vi "configure operation.vi"(7 "tag bus configurable plugin module configuration":refnum<class "PID Module configuration.lvclass">, 8 "error in":errorcluster, 10 "line item in":T1={"Loop ID"="", "Tags"={"Setpoint"="", "Process Variable"="", "Output"=""}, "Gains"={"P"=1.0, "I"=0.01, "D"=0.0}, "Range"={"High"=100.0, "Low"=-100.0}}, 11 "engine configuration":refnum<class "engine configuration.lvclass">) -> (0 "error out":errorcluster, 1 "success":bool, 2 "PID Loop out":T1={"Loop ID"="", "Tags"={"Setpoint"="", "Process Variable"="", "Output"=""}, "Gains"={"P"=1.0, "I"=0.01, "D"=0.0}, "Range"={"High"=100.0, "Low"=-100.0}}, 5 "changed":bool)   [LabVIEW 2014, in "PID Module editor node.lvclass"]
uses:
  PID Module editor node.lvclass
  PID array element.ctl
  <vilib>/NI/Module Execution Interface/Engine Configuration/engine configuration.lvclass
  module/configuration/PID Module configuration.lvclass
panel:
  in  "Range":cluster{"High":dbl, "Low":dbl}
  in  "Gains":cluster{"P":dbl, "I":dbl, "D":dbl}
  in  "Output":i32(listbox)
  in  "Process Variable":i32(listbox)
  out "errors":string
  in  "Setpoint":i32(listbox)
  in  "PID Loop Name":string
  in  "cancel":bool
  in  "ok":bool
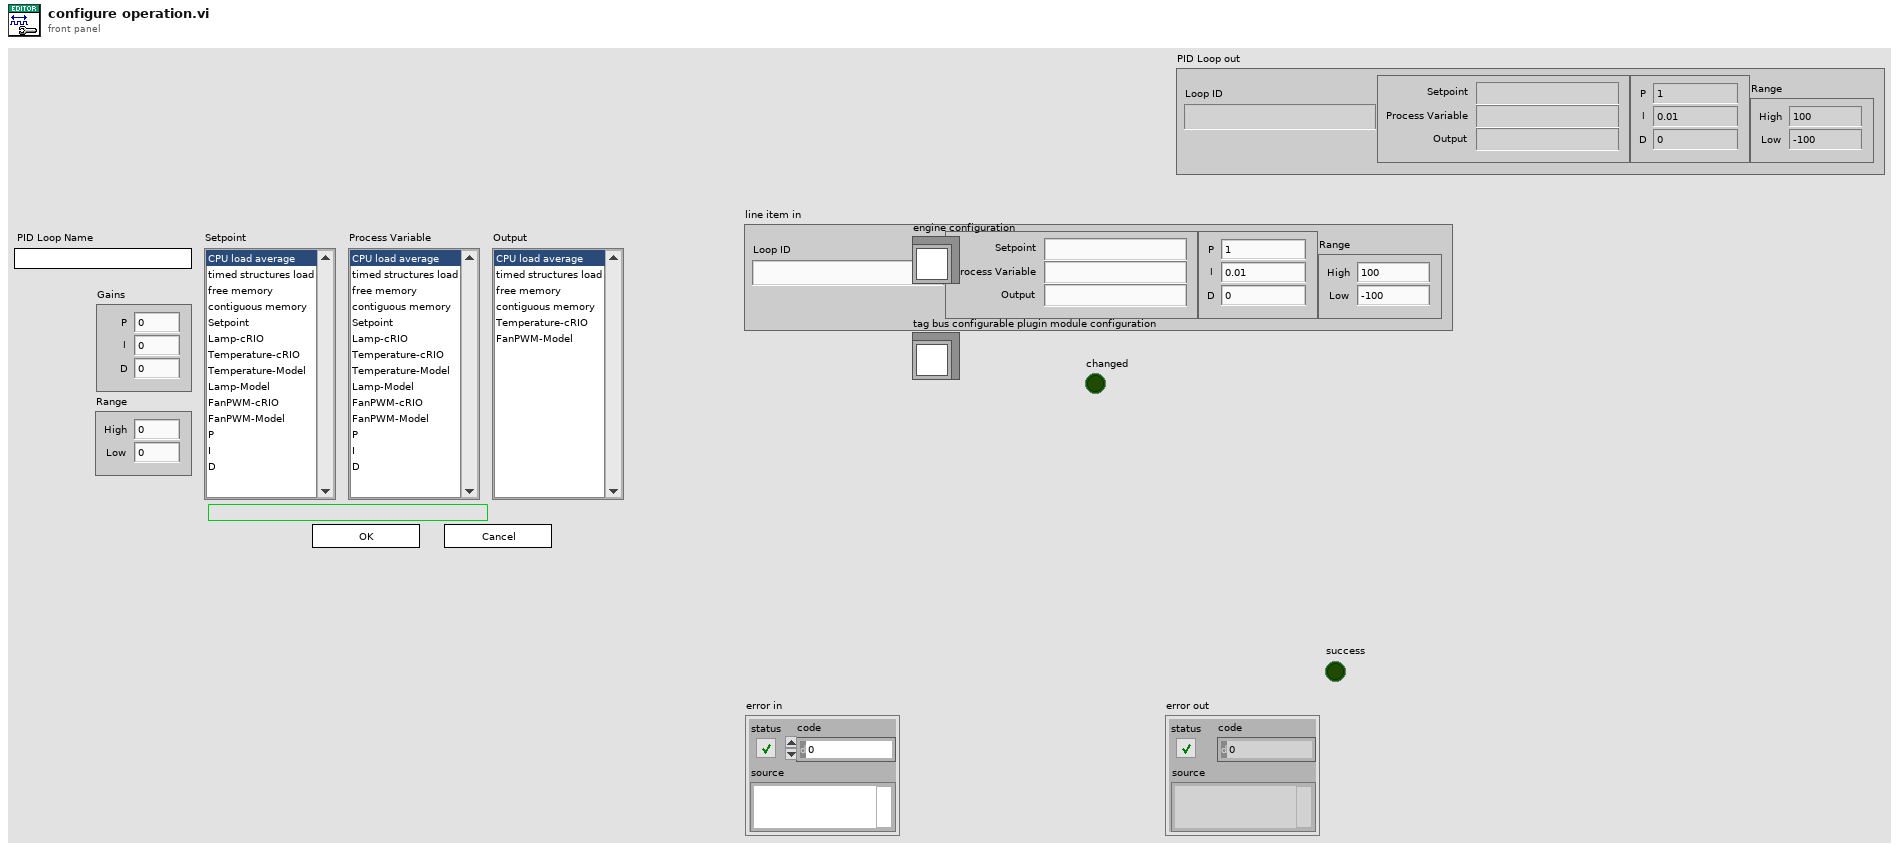
[diagram p1: front panel]
types:
  T1 = typedef "PID Module editor node.lvclass/PID array element.ctl" = cluster{"Loop ID":string, "Tags":cluster{"Setpoint":string, "Process Variable":string, "Output":string}, "Gains":cluster{"P":dbl, "I":dbl, "D":dbl}, "Range":cluster{"High":dbl, "Low":dbl}}
  T2 = enum32{"Invalid", "Standard", "Closed", "Hidden", "Minimized", "Maximized"}
  T3 = enum32{"Invalid", "Default", "Floating", "Floating/Auto-Hide", "Modal"}
  T4 = enum8{"Enabled", "Disabled", "Disabled and Grayed Out"}
  T5 = enum32{"invalid app kind", "Development System", "Run Time System", "Student Edition", "Embedded LabVIEW", "Evaluation", "Custom"}
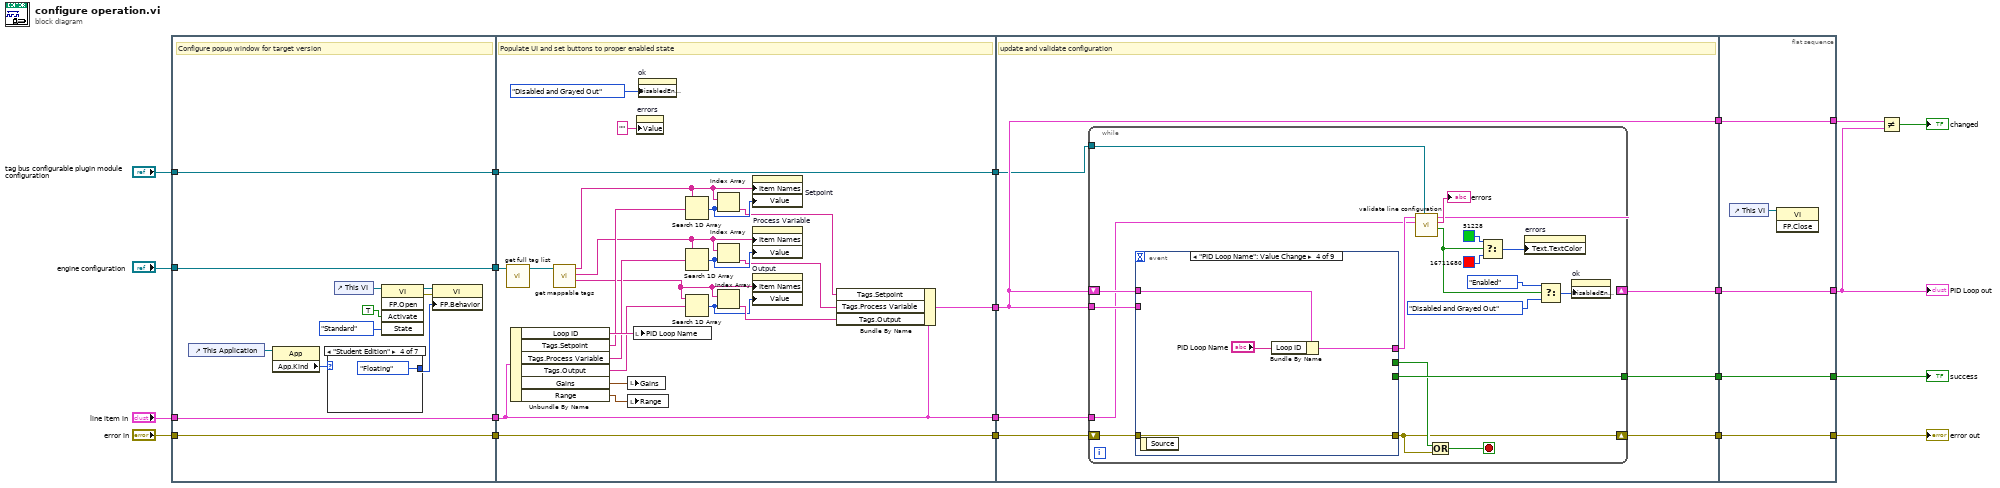
[diagram p0: block diagram]
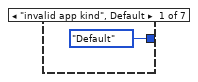
[diagram p2: hidden frame]
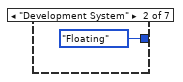
[diagram p3: hidden frame]
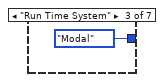
[diagram p4: hidden frame]
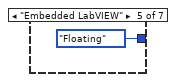
[diagram p5: hidden frame]
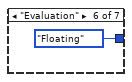
[diagram p6: hidden frame]
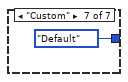
[diagram p7: hidden frame]
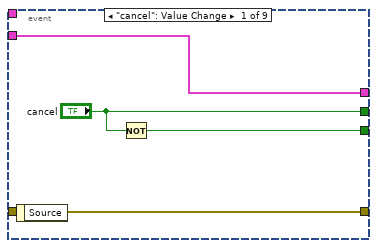
[diagram p8: hidden frame]
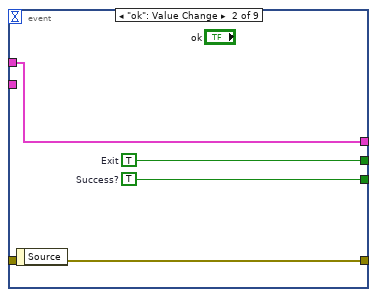
[diagram p9: hidden frame]
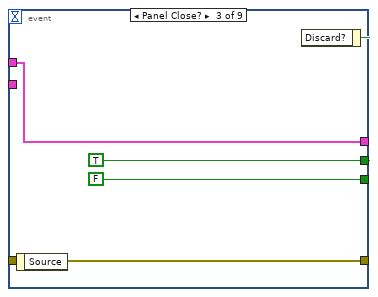
[diagram p10: hidden frame]
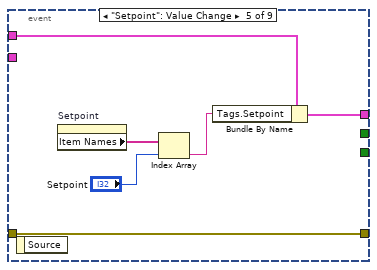
[diagram p11: hidden frame]
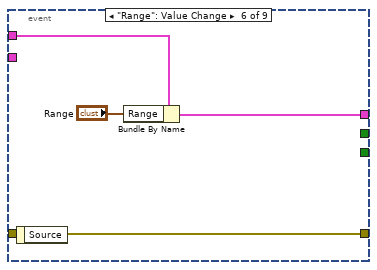
[diagram p12: hidden frame]
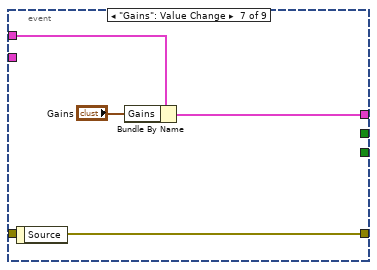
[diagram p13: hidden frame]
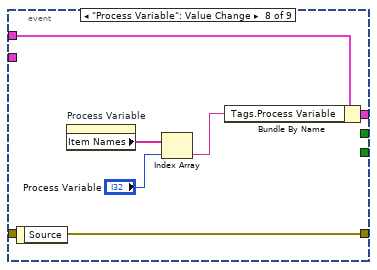
[diagram p14: hidden frame]
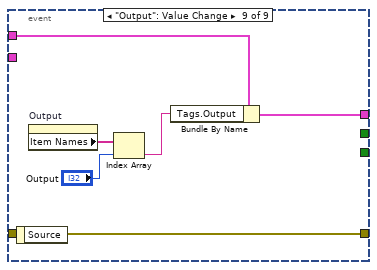
[diagram p15: hidden frame]
diagram:
  n1 = flat-sequence {
    tunnel: "line item in" -> [w32]
    tunnel: "error in" -> [w33]
    tunnel: [w33] -> w10
    tunnel: [w32] -> w9
    tunnel: [w23] -> w7
    tunnel: "engine configuration" -> [w23]
    tunnel: [w22] -> w4
    tunnel: "tag bus configurable plugin module configuration" -> [w22]
    tunnel: w10 -> [w62]
    tunnel: w9 -> [w52]
    tunnel: [w61] -> w8
    tunnel: w7 -> [w47]
    tunnel: [w63] -> w5
    tunnel: w4 -> [w63]
    tunnel: [w62] -> w2
    tunnel: [w52] -> w1
    tunnel: [w69] -> w14
    tunnel: [w68] -> w13
    tunnel: [w67] -> w12
    tunnel: [w66] -> w11
    tunnel: w8 -> [w66]
    tunnel: w5 -> [w65]
    tunnel: w2 -> [w70]
    tunnel: w1 -> [w64]
    tunnel: [w133] -> w15
    tunnel: [w134] -> w18
    tunnel: [w135] -> w19
    tunnel: [w136] -> w20
    tunnel: w14 -> [w136]
    tunnel: w13 -> [w135]
    tunnel: w12 -> [w134]
    tunnel: w11 -> [w133]
    frame #0 {
      # "Configure popup window for target version"
      n2 = control-ref of="This Application"() -> (w26:refnum<vi>)
      n3 = property class="App"(reference=w26) -> ("App.Kind"=w25:T5)  [unwired: 1 in, 2 out]
      n4 = case shown="\"Student Edition\"" w25 {
        tunnel: [T3."Default" ("Front Panel Window:Behavior") T3."Floating" ("Front Panel Window:Behavior") T3."Modal" ("Front Panel Window:Behavior") T3."Floating" ("Front Panel Window:Behavior") T3."Floating" ("Front Panel Window:Behavior") T3."Floating" ("Front Panel Window:Behavior") T3."Default" ("Front Panel Window:Behavior")] -> w24
        frame "invalid app kind", Default {
        }
        frame "Development System" {
        }
        frame "Run Time System" {
        }
        frame "Student Edition" {
        }
        frame "Embedded LabVIEW" {
        }
        frame "Evaluation" {
        }
        frame "Custom" {
        }
      }
      n5 = control-ref of="This VI"() -> (w27:refnum<vi>)
      n6 = invoke class="VI" method="FP.Open"(reference=w27, "Activate"=TRUE ("Activate?"), "State"=T2."Standard") -> (reference out=w30:refnum<vi>, error out=w31:errorcluster)  [unwired: 2 in, 3 out]
      n7 = property class="VI"(reference=w30, error in=w31, "FP.Behavior"=w24) -> ()  [unwired: 2 out]
    }
    frame #1 {
      # "Populate UI and set buttons to proper enabled state"
      n8 = call <vilib>:"get full tag list.vi"("engine configuration in"=w47) -> ("engine configuration out"=w44:refnum<class "engine configuration.lvclass">)  [unwired: 9 in, 1 out]
      n9 = Unbundle By Name(w52) -> ("Loop ID"=w58:string, "Tags.Setpoint"=w55:string, "Tags.Process Variable"=w54:string, "Tags.Output"=w53:string, "Gains"=w56:cluster{"P":dbl, "I":dbl, "D":dbl}, "Range"=w57:cluster{"High":dbl, "Low":dbl})
      n10 = call "get mappable tags.vi"("engine configuration in"=w44) -> ("Output Tags"=w41:string[], "Process Variable Tags"=w42:string[], "Setpoint Tags"=w43:string[])  [unwired: 8 in]
      n11 = local write "Gains"(w56) -> ()
      n12 = local write "Range"(w57) -> ()
      n13 = local write "PID Loop Name"(w58) -> ()
      n14 = property on="errors" class="Str"("Value"="" ("errors")) -> ()  [unwired: 2 in, 2 out]
      n15 = property on="ok" class="Bool"("DisabledEnum"=T4."Disabled and Grayed Out" ("Disabled")) -> ()  [unwired: 2 in, 2 out]
      n16 = Search 1D Array(1D array=w43, element=w55) -> (index of element=w51:i32)  [unwired: 1 in]
      n17 = Search 1D Array(1D array=w42, element=w54) -> (index of element=w50:i32)  [unwired: 1 in]
      n18 = Search 1D Array(1D array=w41, element=w53) -> (index of element=w48:i32)  [unwired: 1 in]
      n19 = Index Array(array=w43, index=w51) -> (element=w46:string)
      n20 = Index Array(array=w42, index=w50) -> (element=w45:string)
      n21 = Index Array(array=w41, index=w48) -> (element=w49:string)
      n22 = property on="Setpoint" class="LstBox (strict)"("Item Names"=w43, "Value"=w51) -> ()  [unwired: 2 in, 2 out]
      n23 = property on="Process Variable" class="LstBox (strict)"("Item Names"=w42, "Value"=w50) -> ()  [unwired: 2 in, 2 out]
      n24 = property on="Output" class="LstBox (strict)"("Item Names"=w41, "Value"=w48) -> ()  [unwired: 2 in, 2 out]
      n25 = Bundle By Name(cluster=w52, "Tags.Setpoint"=w46, "Tags.Process Variable"=w45, "Tags.Output"=w49) -> (w61:T1)
    }
    frame #2 {
      # "update and validate configuration"
      n26 = while {
        shift-right: [w85] -> w68
        shift-left: w70 -> [w89]
        tunnel: [w88] -> w69
        shift-right: [w77] -> w67
        shift-left: w66 -> [w80]
        tunnel: w66 -> [w72]
        tunnel: w65 -> [w81]
        tunnel: w64 -> [w71]
        stop <- w86 stop-if-true
        n27 = event shown="[3] \"PID Loop Name\": Value Change" {
          selector: _ -> [_ _ _ _ _ _ _ _ _]
          dyn-events: _ -> [_ _ _ _ _ _ _ _ _]
          timeout: _ -> [_ _ _ _ _ _ _ _ _]
          tunnel: w89 -> [w93 w97 w101 w105 w106 w115 w119 w120 w127]
          tunnel: [w93 w97 w101 w105 w106 w115 w119 w120 w127] -> w85
          tunnel: [w92 w94 FALSE _ _ _ _ _ _] -> w88
          tunnel: ["cancel" w95 w99 _ _ _ _ _ _] -> w87
          tunnel: w80 -> [_ w96 w98 w103 w111 w114 w118 w124 w131]
          tunnel: [w90 w96 w98 w104 w110 w113 w117 w125 w130] -> w78
          tunnel: w72 -> [w90 _ _ _ _ _ _ _ _]
          event "cancel": Value Change {
            n28 = event-data() -> ()  [unwired: 1 in, 1 out]
            n29 = Not(x="cancel") -> (.not. x?=w92:bool)
          }
          event "ok": Value Change {
            w94 = TRUE  # Success?
            w95 = TRUE  # Exit
            n30 = event-data() -> ()  [unwired: 1 in, 1 out]
          }
          event Panel Close? {
            w99 = TRUE ("cancel")
            n31 = event-data() -> ()  [unwired: 1 in, 1 out]
            n32 = event-data("Discard?"=w99) -> ()  [unwired: 1 in, 1 out]
          }
          event "PID Loop Name": Value Change {
            n33 = event-data() -> ()  [unwired: 1 in, 1 out]
            n34 = Bundle By Name(cluster=w103, "Loop ID"="PID Loop Name") -> (w104:T1)
          }
          event "Setpoint": Value Change {
            n35 = event-data() -> ()  [unwired: 1 in, 1 out]
            n36 = property on="Setpoint" class="LstBox (strict)"() -> ("Item Names"=w109:string[])  [unwired: 2 in, 2 out]
            n37 = Index Array(array=w109, index="Setpoint") -> (element=w107:string)
            n38 = Bundle By Name(cluster=w111, "Tags.Setpoint"=w107) -> (w110:T1)
          }
          event "Range": Value Change {
            n39 = event-data() -> ()  [unwired: 1 in, 1 out]
            n40 = Bundle By Name(cluster=w114, "Range"="Range") -> (w113:T1)
          }
          event "Gains": Value Change {
            n41 = event-data() -> ()  [unwired: 1 in, 1 out]
            n42 = Bundle By Name(cluster=w118, "Gains"="Gains") -> (w117:T1)
          }
          event "Process Variable": Value Change {
            n43 = event-data() -> ()  [unwired: 1 in, 1 out]
            n44 = property on="Process Variable" class="LstBox (strict)"() -> ("Item Names"=w122:string[])  [unwired: 2 in, 2 out]
            n45 = Index Array(array=w122, index="Process Variable") -> (element=w121:string)
            n46 = Bundle By Name(cluster=w124, "Tags.Process Variable"=w121) -> (w125:T1)
          }
          event "Output": Value Change {
            n47 = event-data() -> ()  [unwired: 1 in, 1 out]
            n48 = property on="Output" class="LstBox (strict)"() -> ("Item Names"=w129:string[])  [unwired: 2 in, 2 out]
            n49 = Index Array(array=w129, index="Output") -> (element=w126:string)
            n50 = Bundle By Name(cluster=w131, "Tags.Output"=w126) -> (w130:T1)
          }
        }
        n51 = call "validate line configuration.vi"("module"=w81, "old loop in (optional)"=w71, "new loop in"=w78) -> ("valid?"=w74:bool, "errors"=→"errors":string, "new loop out"=w77:T1)  [unwired: 6 in]
        n52 = Compound Arithmetic op=OR(w87, w85) -> (w86:bool)
        n53 = Select(t=u32 51228, s=w74, f=u32 16711680) -> (s? t:f=w73:u32)
        n54 = property on="errors" class="Str"("Text.TextColor"=w73) -> ()  [unwired: 2 in, 2 out]
        n55 = Select(t=T4."Enabled" ("Disabled"), s=w74, f=T4."Disabled and Grayed Out") -> (s? t:f=w82:T4)
        n56 = property on="ok" class="Bool"("DisabledEnum"=w82) -> ()  [unwired: 2 in, 2 out]
      }
    }
    frame #3 {
      n57 = control-ref of="This VI"() -> (w132:refnum<vi>)
      n58 = invoke class="VI" method="FP.Close"(reference=w132) -> ()  [unwired: 2 in, 3 out]
    }
  }
  n59 = Not Equal?(x=w15, y=w18) -> (x != y?=→"changed":bool)
  "error out" <- w19
  "success" <- w20
  "PID Loop out" <- w18
